vi "Event-Driven State Machine - Main.vi"() -> ()   [LabVIEW 2020]
uses:
  support/State Machine Data.ctl
  support/States.ctl
  <vilib>/Utility/miscctls.llb/LVPointTypeDef.ctl
  <vilib>/DAQmx/read.llb/DAQmx Read (Analog 2D DBL NChan NSamp).vi
  <vilib>/DAQmx/write.llb/DAQmx Write (Analog DBL 1Chan 1Samp).vi
  <vilib>/DAQmx/create/channels.llb/DAQmx Create Channel (AI-Voltage-Basic).vi
  <vilib>/DAQmx/configure/timing.llb/DAQmx Timing (Sample Clock).vi
  <vilib>/DAQmx/miscellaneous.llb/DAQmx Fill In Error Info.vi
  <vilib>/Utility/file.llb/Write Delimited Spreadsheet (DBL).vi
  <vilib>/DAQmx/create/channels.llb/DAQmx Create Channel (AO-Voltage-Basic).vi
panel:
  out "RMS Results Per Channel":dbl[](array[numeric])
  out "Threshold exceeded?":bool
  in  "Acquire":bool
  in  "Samples per channel":i32=100
  in  "Sample Rate":dbl=1000.0
  in  "AI Voltage Channel":tag="PCI-6221/ai0, PCI-6221/ai2:3"
  in  "AO Voltage Channel":tag="PCI-6221/ao0"
  in  "Generate Stimulus":bool
  in  "Threshold (rms)":dbl=1.0
  in  "Clear":bool
  in  "Exit":bool
  out "Graph":dbl[][](graph)
  # "Analysis"
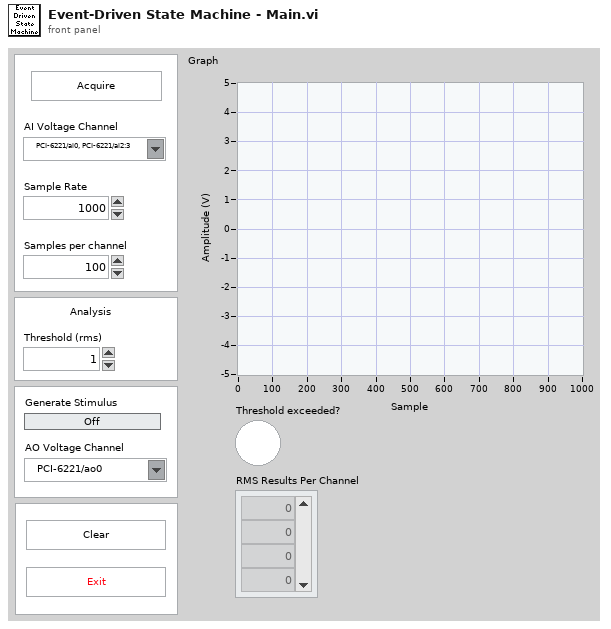
[diagram p1: front panel]
types:
  T1 = typedef "LVPointTypeDef.ctl" = cluster{"Horizontal":i16, "Vertical":i16}
  T2 = typedef "States.ctl" = enum16{"Initialize", "Wait for Event", "Acquire", "Analyze", "Log", "Clear", "Update Stimulus", "Update UI", "Exit"}
  T3 = typedef "State Machine Data.ctl" = cluster{"Acquisition Data":dbl[][], "Stimulus Value":bool}
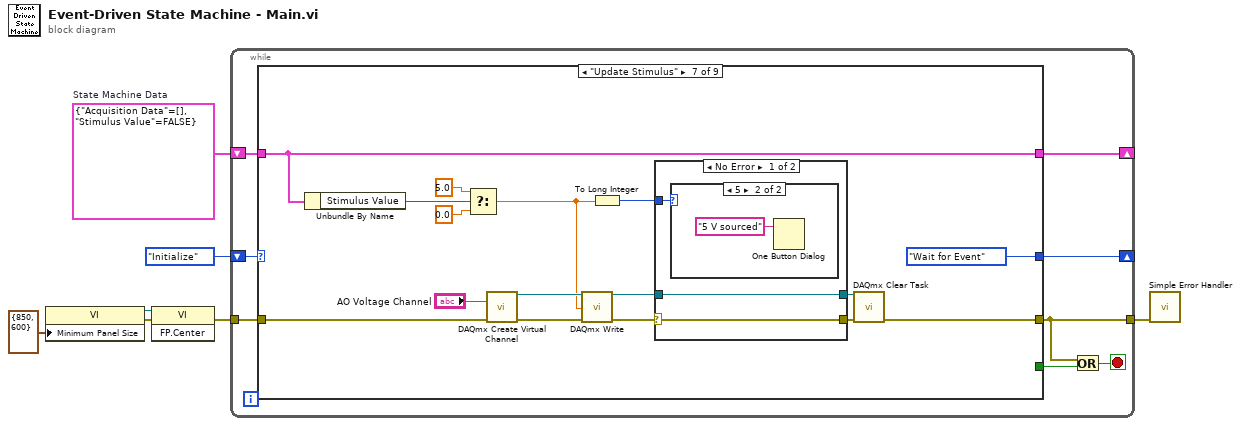
[diagram p0: block diagram]
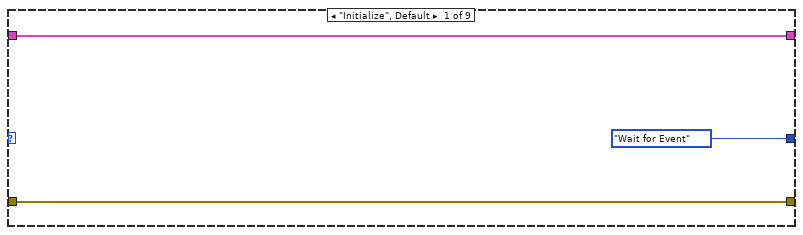
[diagram p2: hidden frame]
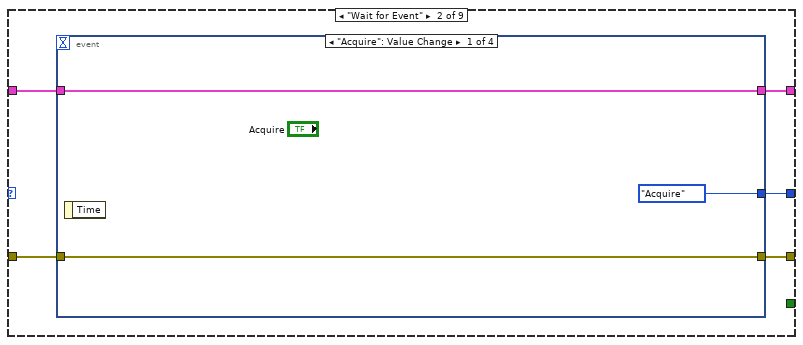
[diagram p3: hidden frame]
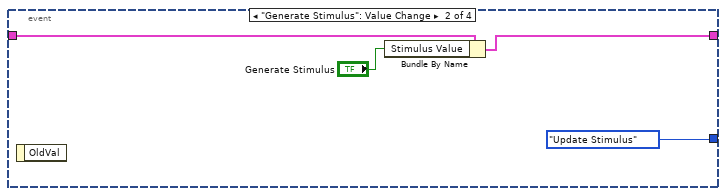
[diagram p4: hidden frame]
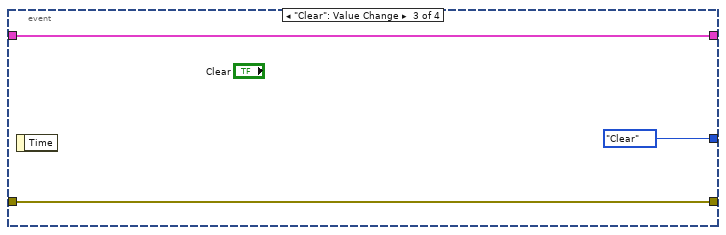
[diagram p5: hidden frame]
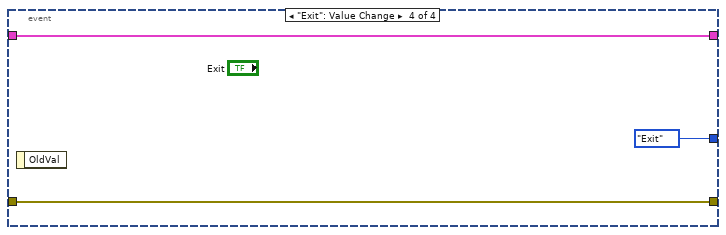
[diagram p6: hidden frame]
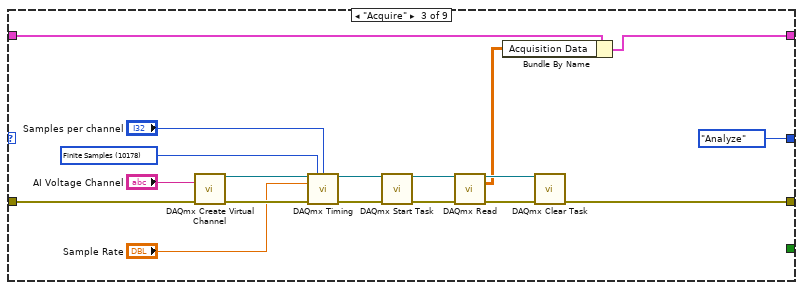
[diagram p7: hidden frame]
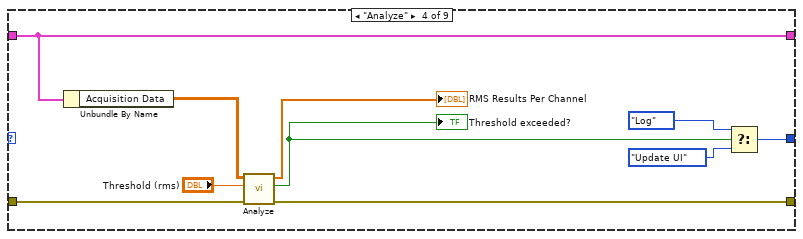
[diagram p8: hidden frame]
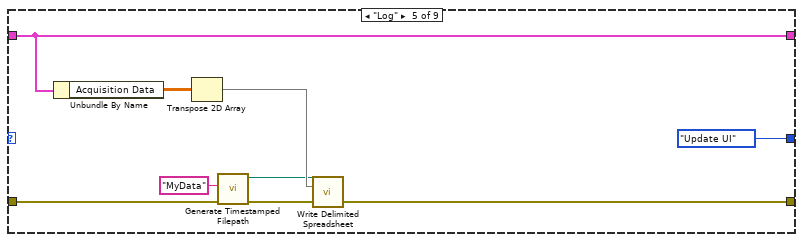
[diagram p9: hidden frame]
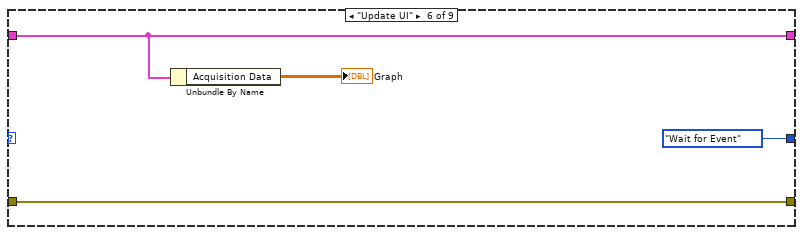
[diagram p10: hidden frame]
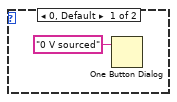
[diagram p11: hidden frame]
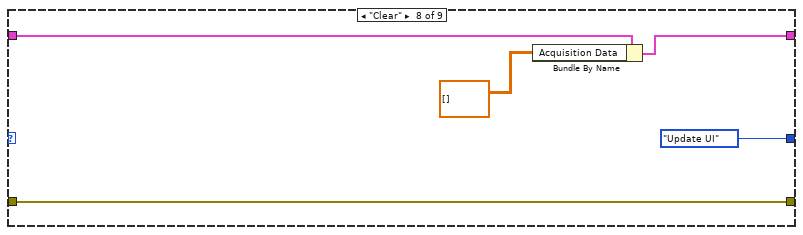
[diagram p13: hidden frame]
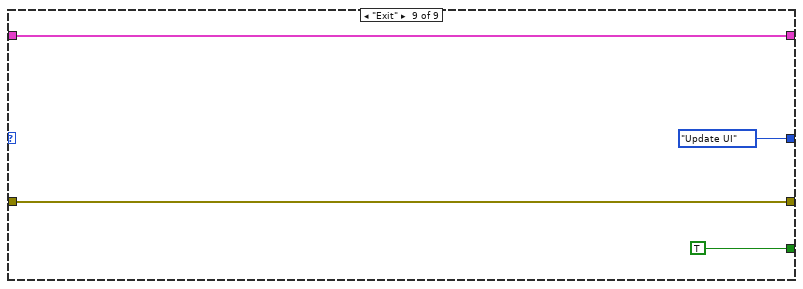
[diagram p14: hidden frame]
diagram:
  w6 = T3 {"Acquisition Data"=[], "Stimulus Value"=FALSE}  # State Machine Data
  n1 = property class="VI"("Minimum Panel Size"=T1 {"Horizontal"=850, "Vertical"=600} ("Front Panel Window:Minimum Size")) -> (reference out=w2:refnum<vi>, error out=w3:errorcluster)  [unwired: 2 in]
  n2 = invoke class="VI" method="FP.Center"(reference=w2, error in=w3) -> (error out=w4:errorcluster)  [unwired: 1 in, 2 out]
  n3 = while {
    shift-right: [w12] -> _
    shift-left: States."Initialize" ("States") -> [w15]
    shift-right: [w13] -> _
    shift-left: w6 -> [w14]
    tunnel: w4 -> [w11]
    tunnel: [w10] -> w5
    stop <- w8 stop-if-true
    n4 = case shown="\"Update Stimulus\"" w15 {
      tunnel: w14 -> [w18 w23 w42 w64 w65 w76 w93 w104 w108]
      tunnel: [w18 w22 w38 w64 w65 w76 w93 w102 w108] -> w13
      tunnel: [States."Wait for Event" ("States") w19 States."Analyze" ("States") w56 States."Update UI" ("States") States."Wait for Event" ("States") States."Wait for Event" ("States") States."Update UI" ("States") States."Update UI" ("States")] -> w12
      tunnel: w11 -> [w16 w21 w54 w61 w71 w77 w87 w105 w109]
      tunnel: [w16 w20 w40 w59 w67 w77 w88 w105 w109] -> w10
      tunnel: [_ _ _ _ _ _ _ _ TRUE] -> w9
      frame "Initialize", Default {
      }
      frame "Wait for Event" {
        n5 = event shown="[0] \"Acquire\": Value Change" {
          selector: _ -> [_ _ _ _]
          dyn-events: _ -> [_ _ _ _]
          timeout: _ -> [_ _ _ _]
          tunnel: w23 -> [w25 w30 w33 w35]
          tunnel: [w25 w29 w33 w35] -> w22
          tunnel: w21 -> [w26 _ w32 w36]
          tunnel: [w26 _ w32 w36] -> w20
          tunnel: [States."Acquire" ("Enum") States."Update Stimulus" ("Enum") States."Clear" ("Enum") States."Exit" ("Enum")] -> w19
          event "Acquire": Value Change {
            n6 = event-data() -> ()  [unwired: 1 in, 1 out]
          }
          event "Generate Stimulus": Value Change {
            n7 = event-data() -> ()  [unwired: 1 in, 1 out]
            n8 = Bundle By Name(cluster=w30, "Stimulus Value"="Generate Stimulus") -> (w29:T3)
          }
          event "Clear": Value Change {
            n9 = event-data() -> ()  [unwired: 1 in, 1 out]
          }
          event "Exit": Value Change {
            n10 = event-data() -> ()  [unwired: 1 in, 1 out]
          }
        }
      }
      frame "Acquire" {
        w50 = 10178 items=["Finite Samples"=10178, "Continuous Samples"=10123, "Hardware Timed Single Point"=12522] ("sample mode")
        n11 = call-poly <vilib>:"DAQmx Create Virtual Channel.vi"("physical channels"="AI Voltage Channel", "error in"=w54) -> ("task out"=w51:refnum<k21>, "error out"=w52:errorcluster)  [unwired: 12 in]
        n12 = call-poly <vilib>:"DAQmx Timing.vi"("task/channels in"=w51, "sample mode"=w50, "samples per channel"="Samples per channel", "rate"="Sample Rate", "error in"=w52) -> ("task out"=w48:refnum<k21>, "error out"=w47:errorcluster)  [unwired: 9 in]
        n13 = call <vilib>:"DAQmx Start Task.vi"("task/channels in"=w48, "error in"=w47) -> ("task out"=w46:refnum<k21>, "error out"=w45:errorcluster)  [unwired: 12 in]
        n14 = call-poly <vilib>:"DAQmx Read.vi"("task/channels in"=w46, "error in"=w45) -> ("task out"=w44:refnum<k21>, "data"=w41:dbl[][], "error out"=w43:errorcluster)  [unwired: 11 in]
        n15 = Bundle By Name(cluster=w42, "Acquisition Data"=w41) -> (w38:T3)
        n16 = call <vilib>:"DAQmx Clear Task.vi"("task in"=w44, "error in"=w43) -> ("error out"=w40:errorcluster)  [unwired: 13 in]
      }
      frame "Analyze" {
        n17 = Unbundle By Name(w64) -> ("Acquisition Data"=w63:dbl[][])
        n18 = call "Analyze.vi"("error in (no error)"=w61, "Threshold (rms)"="Threshold (rms)", "N-Channel Data (2D DBL)"=w63) -> ("error out"=w59:errorcluster, "Threshold Exceeded?"=w55:bool, "N-Channel RMS Results"=→"RMS Results Per Channel":dbl[])  [unwired: 5 in, 1 out]
        "Threshold exceeded?" <- w55
        n19 = Select(t=States."Log" ("States"), s=w55, f=States."Update UI" ("States")) -> (s? t:f=w56:T2)
      }
      frame "Log" {
        n20 = Unbundle By Name(w65) -> ("Acquisition Data"=w73:dbl[][])
        n21 = Transpose 2D Array(2D array=w73) -> (transposed array=w70:dbl[][])
        n22 = call "Generate Timestamped Filepath.vi"("Error In"=w71, "appended filename"="MyData") -> ("Error Out"=w68:errorcluster, "timestamped relative filepath"=w69:path)  [unwired: 8 in]
        n23 = call-poly <vilib>:"Write Delimited Spreadsheet.vi"("file path (dialog if empty)"=w69, "2D data"=w70, "error in (no error)"=w68) -> ("error out"=w67:errorcluster)  [unwired: 11 in, 1 out]
      }
      frame "Update UI" {
        n24 = Unbundle By Name(w76) -> ("Acquisition Data"=→"Graph":dbl[][])
      }
      frame "Update Stimulus" {
        n25 = Unbundle By Name(w93) -> ("Stimulus Value"=w84:bool)
        n26 = Select(t=5.0, s=w84, f=0.0) -> (s? t:f=w83:dbl)
        n27 = call-poly <vilib>:"DAQmx Create Virtual Channel.vi"("physical channels"="AO Voltage Channel", "error in"=w87) -> ("task out"=w90:refnum<k21>, "error out"=w89:errorcluster)  [unwired: 12 in]
        n28 = call-poly <vilib>:"DAQmx Write.vi"("task/channels in"=w90, "data"=w83, "error in"=w89) -> ("task out"=w80:refnum<k21>, "error out"=w81:errorcluster)  [unwired: 10 in, 1 out]
        n29 = To Long Integer(number=w83) -> (32bit integer=w82:i32)
        n30 = case shown="No Error" w81 {
          selector: w81 -> [w94 w99]
          tunnel: w82 -> [w96 _]
          tunnel: w80 -> [w95 w100]
          tunnel: [w95 w100] -> w79
          tunnel: [w94 w99] -> w78
          frame No Error {
            n31 = case shown="5" w96 {
              frame 0, Default {
                n32 = One Button Dialog(message="0 V sourced") -> ()  [unwired: 1 in, 1 out]
              }
              frame 5 {
                n33 = One Button Dialog(message="5 V sourced") -> ()  [unwired: 1 in, 1 out]
              }
            }
          }
          frame Error {
          }
        }
        n34 = call <vilib>:"DAQmx Clear Task.vi"("task in"=w79, "error in"=w78) -> ("error out"=w88:errorcluster)  [unwired: 13 in]
      }
      frame "Clear" {
        n35 = Bundle By Name(cluster=w104, "Acquisition Data"=dbl[][] []) -> (w102:T3)
      }
      frame "Exit" {
      }
    }
    n36 = Or(x=w10, y=w9) -> (x .or. y?=w8:bool)
  }
  n37 = call <vilib>:"Simple Error Handler.vi"("error in (no error)"=w5) -> ()  [unwired: 4 in, 5 out]
